vi "WiFi HttpGET_NTPtime.vi"   [LabVIEW 2014]
uses:
  <vilib>/Aledyne-TSXperts/Arduino Compatible Compiler for LabVIEW/Code Generator/Arduino APIs/Digital/PinDirection.ctl
  QwaveSys_ESP8266/QwaveSys_ESP8266.lvlib
  <vilib>/Aledyne-TSXperts/Arduino Compatible Compiler for LabVIEW/Arduino Compatible Compiler for LabVIEW.lvlib
types:
  T1 = typedef "Arduino Compatible Compiler for LabVIEW.lvlib/PinDirection.ctl" = enum16{" INPUT", "OUTPUT", " INPUT_PULLUP"}
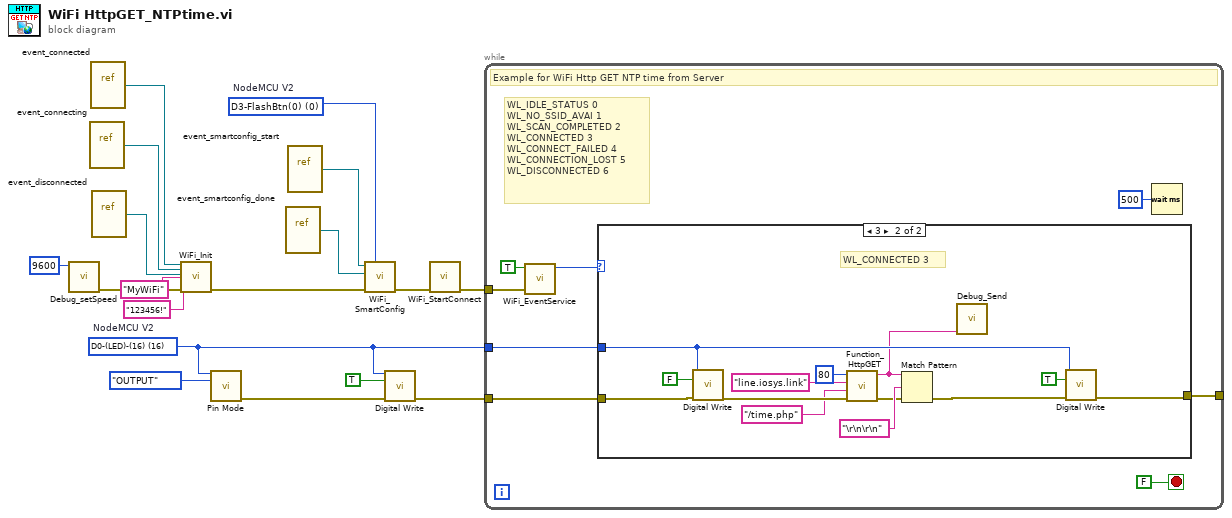
[diagram p0: block diagram]
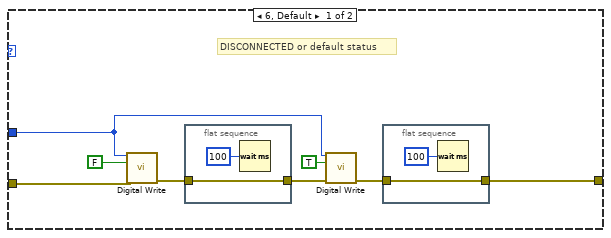
[diagram p2: hidden frame]
diagram:
  w4 = u8 16 items=["D0-(LED)-(16)"=16, "D1-SCL(5)"=5, "D2-SDA(4)"=4, "D3-FlashBtn(0)"=0, "D4-(2)"=2, "D5-SCK(14)"=14, "D6-MISO(12)"=12, "D7-MOSI(13)"=13, "D8-SS(15)"=15, "D9-TX(3)"=3, "D10-RX(1)"=1, "ADC0,(17)"=17]  # NodeMCU V2
  w3 = u8 0 items=["D0-(LED)-(16)"=16, "D1-SCL(5)"=5, "D2-SDA(4)"=4, "D3-FlashBtn(0)"=0, "D4-(2)"=2, "D5-SCK(14)"=14, "D6-MISO(12)"=12, "D7-MOSI(13)"=13, "D8-SS(15)"=15, "D9-TX(3)"=3, "D10-RX(1)"=1, "ADC0,(17)"=17]  # NodeMCU V2
  n1 = call "Debug_setSpeed.vi"("Speed"=u32 9600) -> ("error out"=w10:errorcluster)  [unwired: 10 in]
  n2 = vi-ref "event_connecting.vi"() -> (w15:refnum<vi>)
  n3 = vi-ref "event_connected.vi"() -> (w14:refnum<vi>)
  n4 = vi-ref "event_disconnected.vi"() -> (w13:refnum<vi>)
  n5 = call "WiFi_Init.vi"("connected"=w14, "connecting"=w15, "disconnected"=w13, "SSID"="MyWiFi", "PASSPHARSE"="123456!", "error in (no error)"=w10) -> ("error out"=w18:errorcluster)  [unwired: 9 in]
  n6 = call <vilib>:"Pin Mode.vi"("pin"=w4, "direction"=PinDirection."OUTPUT" ("Direction")) -> ("error out"=w6:errorcluster)  [unwired: 13 in]
  n7 = vi-ref "event_smartconfig_done.vi"() -> (w11:refnum<vi>)
  n8 = vi-ref "event_smartconfig_start.vi"() -> (w12:refnum<vi>)
  n9 = call "WiFi_SmartConfig.vi"("Smart Config Enter Pin"=w3, "error in (no error)"=w18, "smartconfig_done"=w11, "smartconfig_start"=w12) -> ("error out"=w17:errorcluster)  [unwired: 7 in]
  n10 = call <vilib>:"Digital Write.vi"("pin"=w4, "state"=TRUE, "error in (no error)"=w6) -> ("error out"=w5:errorcluster)  [unwired: 12 in]
  n11 = call "WiFi_StartConnect.vi"("error in (no error)"=w17) -> ("error out"=w16:errorcluster)  [unwired: 10 in]
  n12 = while {
    tunnel: w16 -> [w25]
    tunnel: w5 -> [w21]
    tunnel: w4 -> [w20]
    tunnel: [w19] -> _
    stop <- FALSE stop-if-true
    # "WL_IDLE_STATUS\t0\nWL_NO_SSID_AVAI\t1\nWL_SCAN_COMPLETED\t2\nWL_CONNECTED\t3\nWL_CONNECT_FAILED\t4\nWL_CONNECTION_LOST\t5\nWL_DISCONNECTED\t6"
    # "Example for WiFi Http GET NTP time from Server"
    n13 = call "WiFi_EventService.vi"("error in (no error)"=w25, "wait for connected (True)"=TRUE) -> ("Status"=w22:u16)  [unwired: 8 in, 1 out]
    n14 = case shown="3" w22 {
      tunnel: w21 -> [w29 w44]
      tunnel: w20 -> [w28 w43]
      tunnel: [w27 w41] -> w19
      frame 6, Default {
        # "DISCONNECTED or default status"
        n15 = call <vilib>:"Digital Write.vi"("pin"=w28, "state"=FALSE, "error in (no error)"=w29) -> ("error out"=w30:errorcluster)  [unwired: 12 in]
        n16 = flat-sequence {
          tunnel: w30 -> [w37]
          tunnel: [w37] -> w31
          frame #0 {
            n17 = Wait (ms)(milliseconds to wait=u32 100) -> ()  [unwired: 1 out]
          }
        }
        n18 = call <vilib>:"Digital Write.vi"("pin"=w28, "state"=TRUE, "error in (no error)"=w31) -> ("error out"=w34:errorcluster)  [unwired: 12 in]
        n19 = flat-sequence {
          tunnel: w34 -> [w35]
          tunnel: [w35] -> w27
          frame #0 {
            n20 = Wait (ms)(milliseconds to wait=u32 100) -> ()  [unwired: 1 out]
          }
        }
      }
      frame 3 {
        # "WL_CONNECTED\t3"
        n21 = call <vilib>:"Digital Write.vi"("pin"=w43, "state"=FALSE, "error in (no error)"=w44) -> ("error out"=w47:errorcluster)  [unwired: 12 in]
        n22 = call "Function_HttpGET.vi"("error in (no error)"=w47, "URI"="/time.php", "Host"="line.iosys.link", "Port"=i8 80) -> ("error out"=w40:errorcluster, "Results"=w39:string)  [unwired: 6 in]
        n23 = Match Pattern(string=w39, regular expression="\r\n\r\n") -> ()  [unwired: 1 in, 4 out]
        n24 = call "Debug_Send.vi"("DATA"=w39) -> ()  [unwired: 11 in]
        n25 = call <vilib>:"Digital Write.vi"("pin"=w43, "state"=TRUE, "error in (no error)"=w40) -> ("error out"=w41:errorcluster)  [unwired: 12 in]
      }
    }
    n26 = Wait (ms)(milliseconds to wait=u32 500) -> ()  [unwired: 1 out]
  }
